vi "Read Element of Headers.vi"(8 "error in (no error)":errorcluster, 10 "index":i32, 11 "Request in":refnum<class "Request.lvclass">) -> (0 "error out":errorcluster, 2 "Header":cluster{"Name":string, "Value":string}, 3 "Request out":refnum<class "Request.lvclass">)   [LabVIEW 2016, in "Request.lvclass"]
uses:
  Request/Request.lvclass
  Request/Request.lvclass/Request.ctl
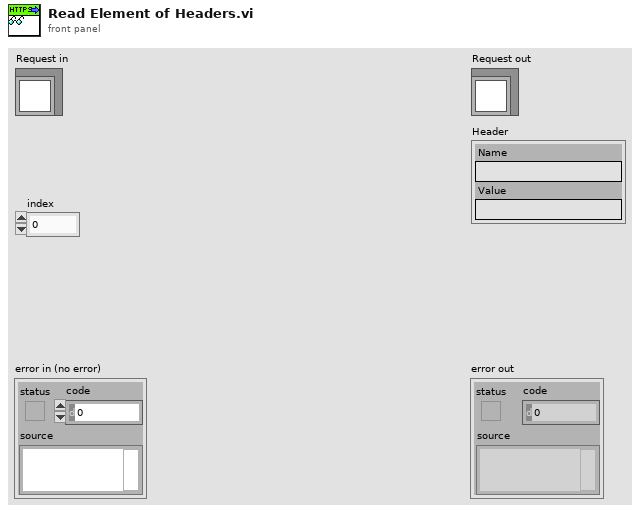
[diagram p1: front panel]
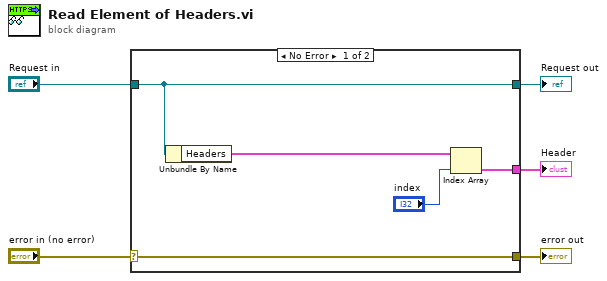
[diagram p0: block diagram]
diagram:
  n1 = case shown="No Error" "error in (no error)" {
    selector: "error in (no error)" -> [w10 w11]
    tunnel: [w10 w11] -> w4
    tunnel: [w9 w12] -> w2
    tunnel: "Request in" -> [w9 w12]
    tunnel: [w6 _] -> w1
    frame No Error {
      n2 = Unbundle By Name(w9) -> ("Headers"=w8:cluster{"Name":string, "Value":string}[])
      n3 = Index Array(array=w8, index="index") -> (element=w6:cluster{"Name":string, "Value":string})
    }
    frame Error {
    }
  }
  "error out" <- w4
  "Request out" <- w2
  "Header" <- w1
